vi "Main.vi"() -> ()   [LabVIEW 2017]
uses:
  <vilib>/Utility/file.llb/Write Delimited Spreadsheet (string).vi
  TCP/TCP Engine/SubVIs/SubVI - Global.vi
  TCP/TCP Engine/Controls/RT- Queue States.ctl
  TCP/TCP Engine/TCP/TCP - Driver Control.ctl
  TCP/TCP Engine/TCP/TCP - Signal Names.ctl
  TCP/TCP Engine/TCP/TCP - Signals.ctl
  Global_simulator.vi
panel:
  out "Datalog Interval":dbl
  out "Test Running":bool
  out "Elapsed Time":dbl format="%#.2g"
  out "File Path":path
  out "Test Running":bool
  out "Test Start":u32
  in  "error in (no error)":errorcluster
  out "Data 2":u32
  out "Data 1":u32
  in  "DI 64":bool
  in  "DI 63":bool
  in  "DI 62":bool
  in  "DI 61":bool
  in  "DI 60":bool
  in  "DI 59":bool
  in  "DI 58":bool
  in  "DI 57":bool
  in  "DI 56":bool
  in  "DI 55":bool
  in  "DI 54":bool
  in  "DI 53":bool
  in  "DI 52":bool
  in  "DI 51":bool
  in  "DI 50":bool
  in  "DI 49":bool
  in  "DI 48":bool
  in  "DI 47":bool
  in  "DI 46":bool
  in  "DI 45":bool
  in  "DI 44":bool
  in  "DI 43":bool
  in  "DI 42":bool
  in  "DI 41":bool
  in  "DI 40":bool
  in  "DI 39":bool
  in  "DI 38":bool
  in  "DI 37":bool
  in  "DI 36":bool
  in  "DI 35":bool
  in  "DI 34":bool
  in  "DI 33":bool
  in  "DI 32":bool
  in  "DI 31":bool
  in  "DI 30":bool
  in  "DI 29":bool
  in  "DI 28":bool
  in  "DI 27":bool
  in  "DI 26":bool
  in  "DI 25":bool
  in  "DI 24":bool
  in  "DI 23":bool
  in  "DI 22":bool
  in  "DI 21":bool
  in  "DI 20":bool
  in  "DI 19":bool
  in  "DI 18":bool
  in  "DI 17":bool
  in  "DI 16":bool
  in  "DI 15":bool
  in  "DI 14":bool
  in  "DI 13":bool
  in  "DI 12":bool
  in  "DI 11":bool
  in  "DI 10":bool
  in  "DI 9":bool
  in  "DI 8":bool
  in  "DI 7":bool
  in  "DI 6":bool
  in  "DI 5":bool
  in  "DI 4":bool
  in  "DI 3":bool
  in  "DI 2":bool
  in  "DI 1":bool
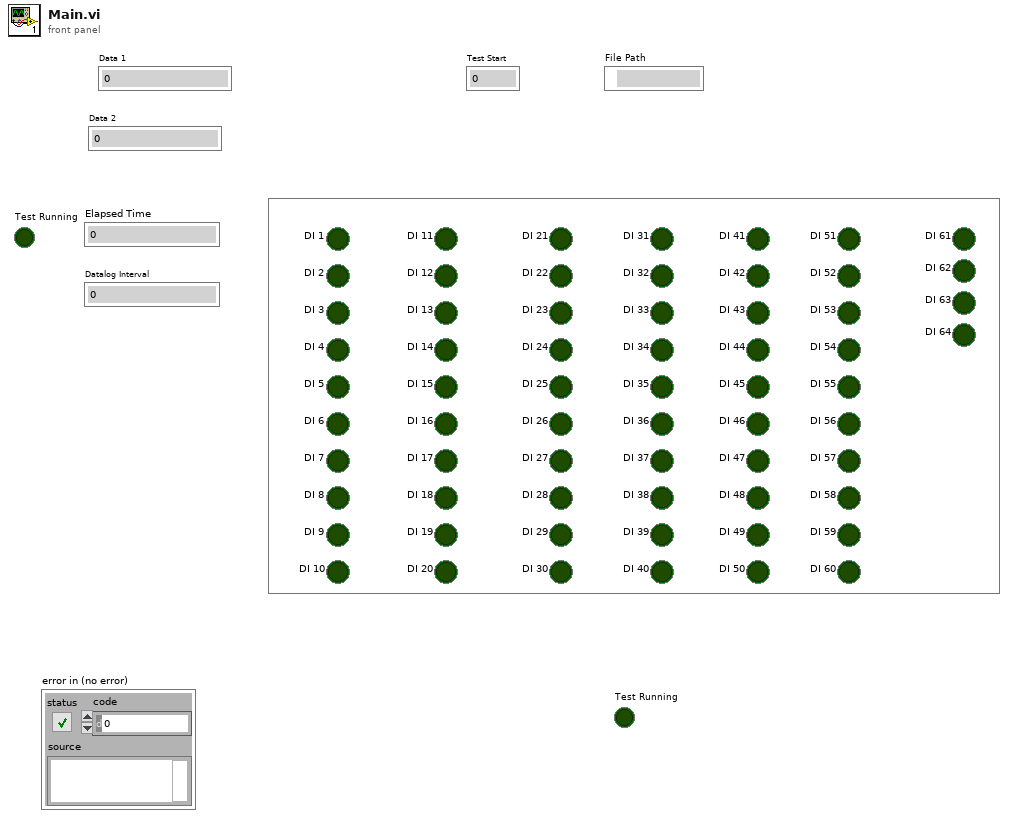
[diagram p1: front panel]
types:
  T1 = cluster{"Data 1":u32, "Data 2":u32, "Boolean Data1":bool[], "Boolean Data 2":bool[]}
  T2 = typedef "TCP - Signals.ctl" = cluster{"Signal":T3, "Value":bool, "Data":variant}
  T3 = typedef "TCP - Signal Names.ctl" = enum16{"Test Running", "Update Sensor Data", "Start Test", "Test Started", "Sequence Complete", "Seuence Aborted", "Abort Test", "Test Settings Updated", "Log Path", "Update Manual Values", "Start Aux Logging", "Aux Log Started", "Stop Aux Logging", "Aux Log Stopped", "Set Dyno Config", "Get PID Values", "Reset Emergency", "Copy Log File", "Download Files", "Send Test Details"}
  T4 = typedef "TCP - Driver Control.ctl" = enum16{"Test Settings", "Boolean Commands", "Test Results", "Send Test Details"}
  T5 = typedef "RT- Queue States.ctl" = enum16{"Initialize", "Enqueue", "Enqueue Priority", "Dequeue", "Flush", "Destroy"}
  T6 = cluster{"Histogram Data":i32[], "Sensor Data":i32[], "File Path":path}
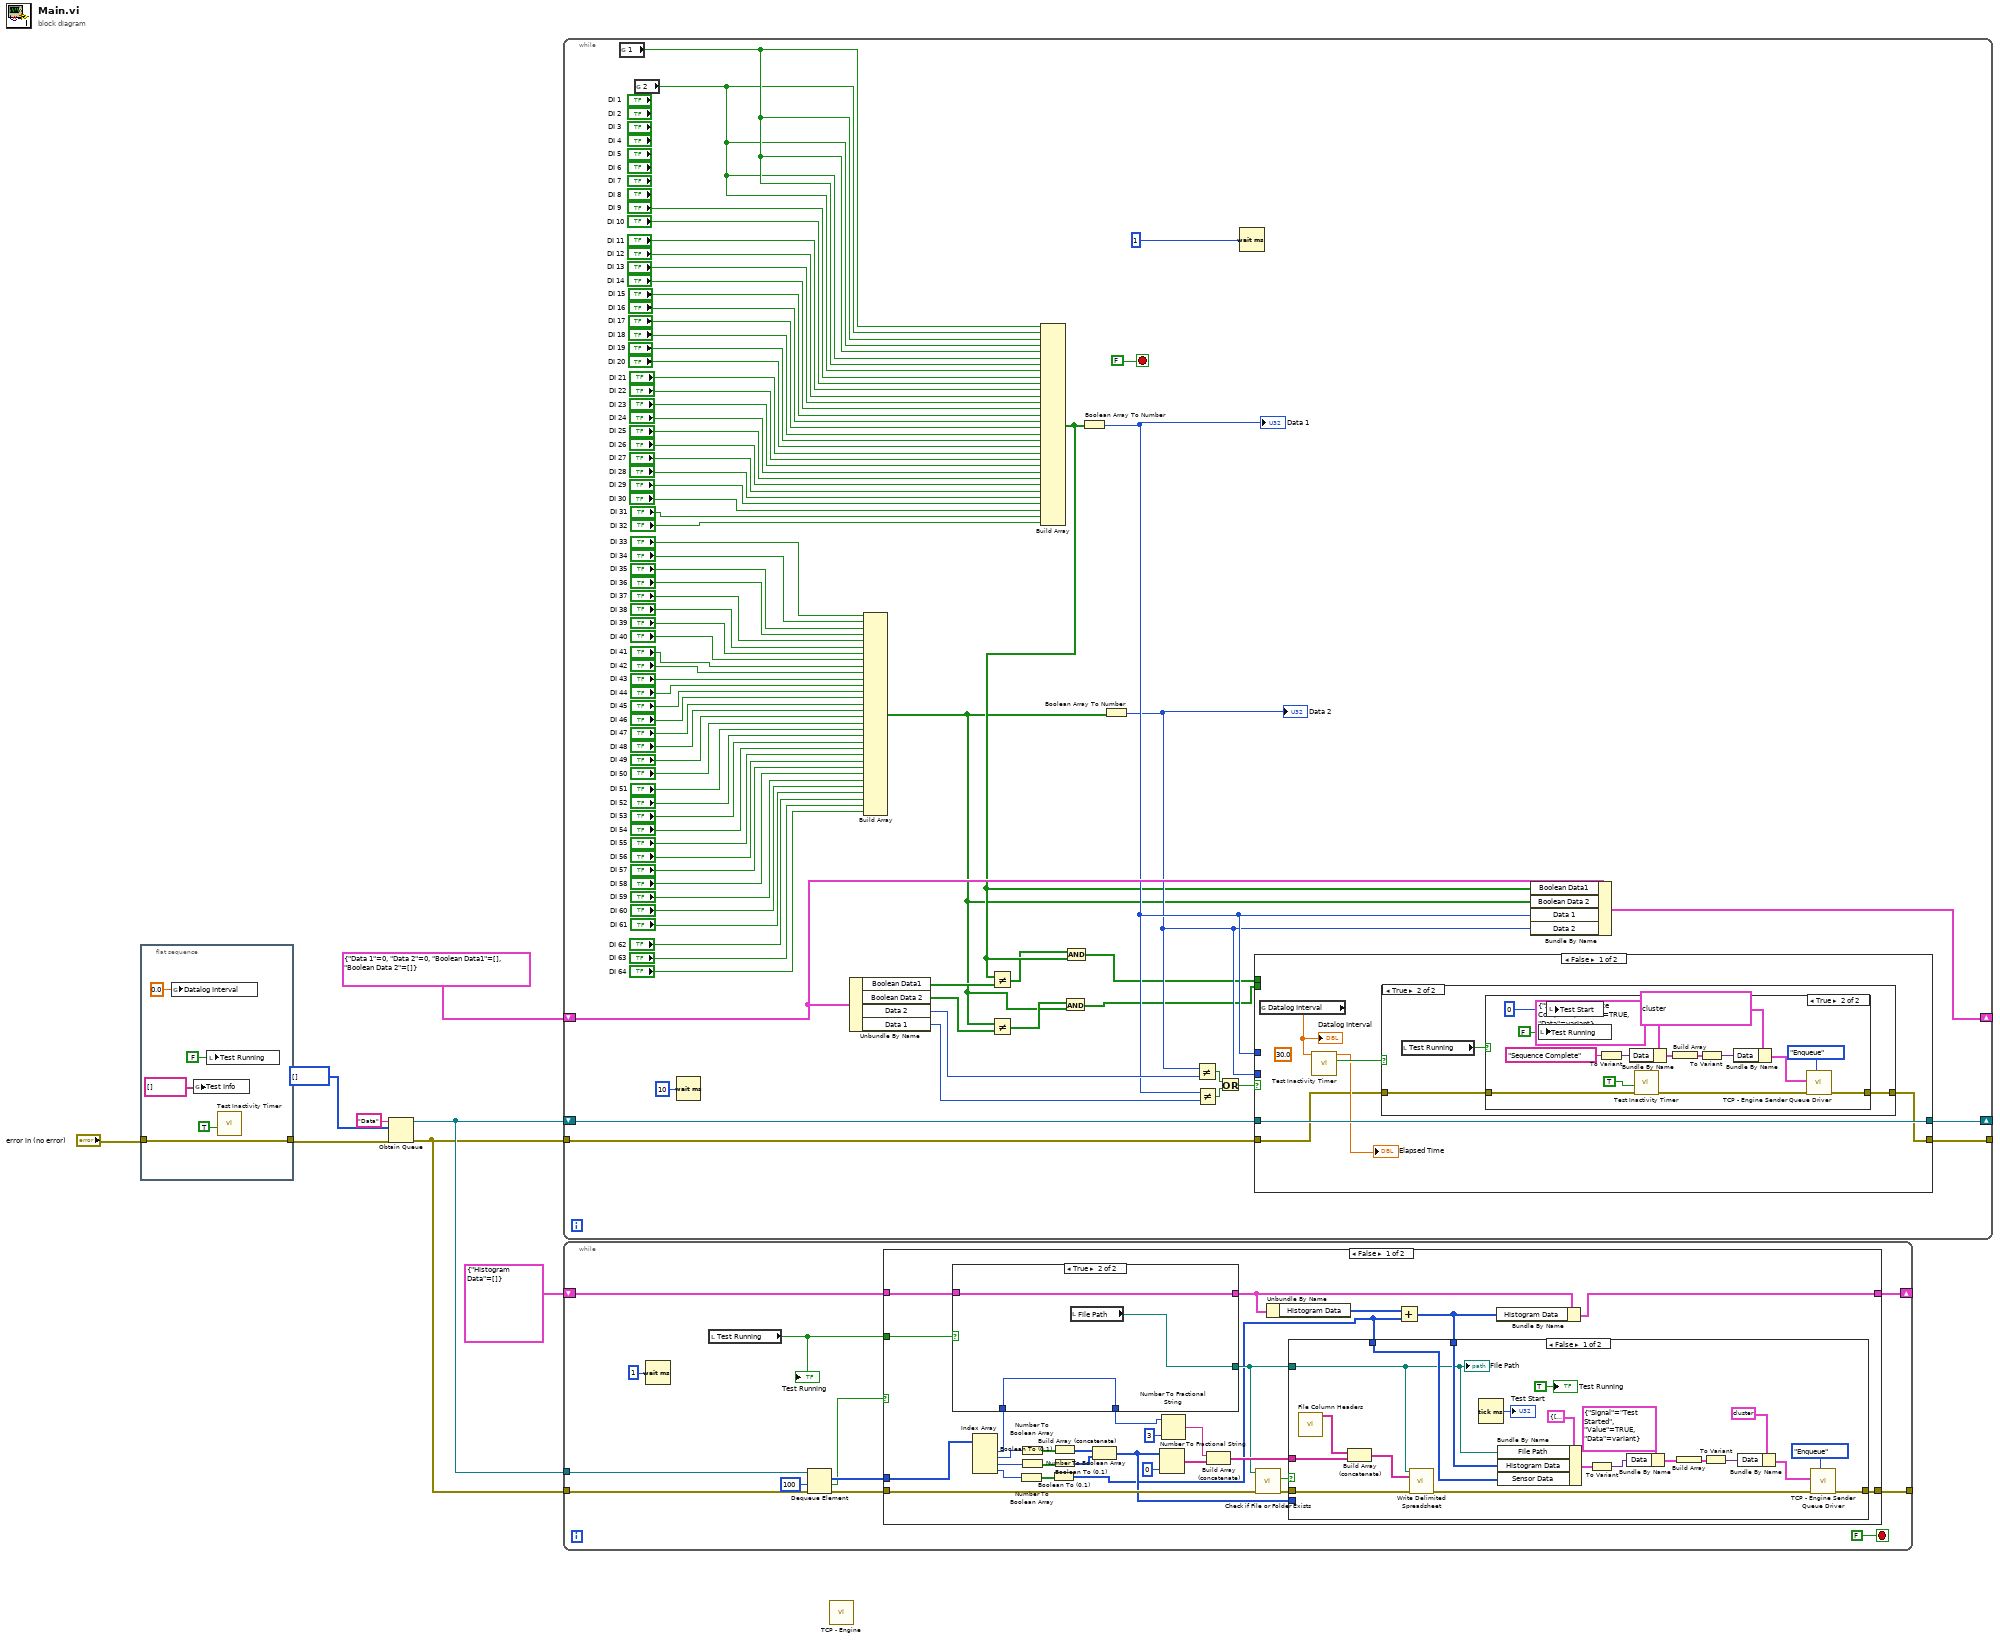
[diagram p0: block diagram]
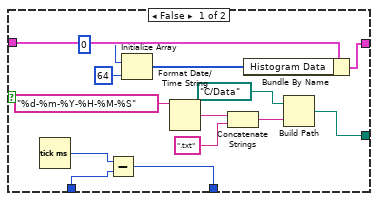
[diagram p2: hidden frame]
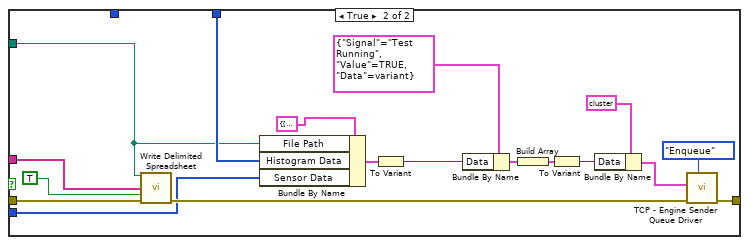
[diagram p3: hidden frame]
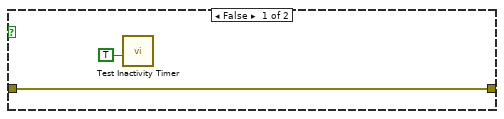
[diagram p6: hidden frame]
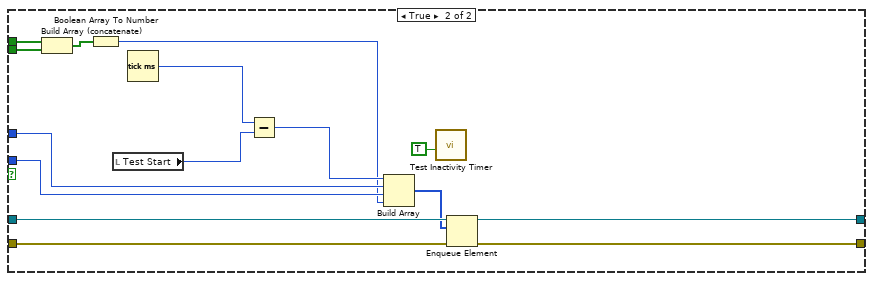
[diagram p7: hidden frame]
diagram:
  n1 = flat-sequence {
    tunnel: [w13] -> w2
    tunnel: "error in (no error)" -> [w13]
    frame #0 {
      n2 = global write "SubVI - Global.vi" "Datalog Interval"(0.0 ("Datalog Interval")) -> ()
      n3 = global write "SubVI - Global.vi" "Test Info"(string[] [] ("Test Info")) -> ()
      n4 = local write "Test Running"(FALSE ("Test Running")) -> ()
      n5 = call "Test Inactivity Timer.vi"("Reset"=TRUE) -> ()  [unwired: 8 in, 3 out]
    }
  }
  n6 = Obtain Queue(name (unnamed)="Data", element data type=u32[] [], error in (no error)=w2) -> (queue out=w5:refnum<queue>, error out=w4:errorcluster)  [unwired: 2 in, 1 out]
  n7 = while {
    shift-right: [w35] -> _
    shift-left: w5 -> [w37]
    tunnel: w4 -> [w36]
    tunnel: [w34] -> _
    shift-right: [w25] -> _
    shift-left: T1 {"Data 1"=0, "Data 2"=0, "Boolean Data1"=[], "Boolean Data 2"=[]} -> [w28]
    stop <- FALSE stop-if-true
    n8 = global read "Global_simulator.vi" "1"() -> (w15:bool)
    n9 = global read "Global_simulator.vi" "2"() -> (w14:bool)
    n10 = Wait (ms)(milliseconds to wait=u32 10) -> ()  [unwired: 1 out]
    n11 = Unbundle By Name(w28) -> ("Boolean Data1"=w23:bool[], "Boolean Data 2"=w22:bool[], "Data 2"=w32:u32, "Data 1"=w33:u32)
    n12 = Build Array("DI 33", "DI 34", "DI 35", "DI 36", "DI 37", "DI 38", "DI 39", "DI 40", "DI 41", "DI 42", "DI 43", "DI 44", "DI 45", "DI 46", "DI 47", "DI 48", "DI 49", "DI 50", "DI 51", "DI 52", "DI 53", "DI 54", "DI 55", "DI 56", "DI 57", "DI 58", "DI 59", "DI 60", "DI 61", "DI 62", "DI 63", "DI 64") -> (w18:bool[])
    n13 = Not Equal?(x=w18, y=w22) -> (x != y?=w21:bool[])
    n14 = Build Array(w15, w14, w15, w14, w15, w14, w15, w14, "DI 9", "DI 10", "DI 11", "DI 12", "DI 13", "DI 14", "DI 15", "DI 16", "DI 17", "DI 18", "DI 19", "DI 20", "DI 21", "DI 22", "DI 23", "DI 24", "DI 25", "DI 26", "DI 27", "DI 28", "DI 29", "DI 30", "DI 31", "DI 32") -> (w19:bool[])
    n15 = Not Equal?(x=w19, y=w23) -> (x != y?=w17:bool[])
    n16 = And(x=w21, y=w18) -> (x .and. y?=w20:bool[])
    n17 = And(x=w17, y=w19) -> (x .and. y?=w16:bool[])
    n18 = Boolean Array To Number(Boolean array=w19) -> (number=w27:u32)
    "Data 1" <- w27
    n19 = Boolean Array To Number(Boolean array=w18) -> (number=w26:u32)
    "Data 2" <- w26
    n20 = Not Equal?(x=w26, y=w32) -> (x != y?=w31:bool)
    n21 = Not Equal?(x=w27, y=w33) -> (x != y?=w30:bool)
    n22 = Or(x=w31, y=w30) -> (x .or. y?=w29:bool)
    n23 = Wait (ms)(milliseconds to wait=u32 1) -> ()  [unwired: 1 out]
    n24 = case shown="False" w29 {
      tunnel: w37 -> [w101 w137]
      tunnel: w36 -> [w97 w136]
      tunnel: [w101 w135] -> w35
      tunnel: [w98 w134] -> w34
      tunnel: w27 -> [_ w130]
      tunnel: w26 -> [_ w129]
      tunnel: w16 -> [_ w126]
      tunnel: w20 -> [_ w125]
      frame False {
        (unwired) 30.0 ("Target Time")
        n25 = global read "SubVI - Global.vi" "Datalog Interval"() -> (w96:dbl)
        "Datalog Interval" <- w96
        n26 = call "Test Inactivity Timer.vi"("Target Time"=w96) -> ("Time Elapsed"=w100:bool, "Elapsed Time"=→"Elapsed Time":dbl)  [unwired: 8 in, 1 out]
        n27 = case shown="True" w100 {
          tunnel: [w102 w105] -> w98
          tunnel: w97 -> [w102 w104]
          frame False {
          }
          frame True {
            n28 = local read "Test Running"() -> (w103:bool)
            n29 = case shown="True" w103 {
              tunnel: [w107 w111] -> w105
              tunnel: w104 -> [w107 w110]
              frame False {
                n30 = call "Test Inactivity Timer.vi"("Reset"=TRUE) -> ()  [unwired: 8 in, 3 out]
              }
              frame True {
                n31 = local write "Test Running"(FALSE ("Test Running")) -> ()
                n32 = local write "Test Start"(u32 0 ("Test Start")) -> ()
                n33 = To Variant(anything="Sequence Complete") -> (Variant=w108:variant)
                n34 = Bundle By Name(cluster=T2 {"Signal"=enum."Sequence Complete", "Value"=TRUE, "Data"=variant}, "Data"=w108) -> (w117:T2)
                n35 = call "Test Inactivity Timer.vi"("error in (no error)"=w110, "Reset"=TRUE) -> ("error out"=w112:errorcluster)  [unwired: 7 in, 2 out]
                n36 = Build Array(w117) -> (w119:T2[])
                n37 = To Variant(anything=w119) -> (Variant=w118:variant)
                n38 = Bundle By Name(cluster=cluster{"Data":variant, "State":T4} {"Data"=variant, "State"=enum."Boolean Commands"} ("Element In"), "Data"=w118) -> (w113:cluster{"Data":variant, "State":T4})
                n39 = call "TCP - Engine Sender Queue Driver.vi"("Cases"=RT-_Queue_States."Enqueue", "error in (no error)"=w112, "Element In"=w113) -> ("error out"=w111:errorcluster)  [unwired: 6 in, 2 out]
              }
            }
          }
        }
      }
      frame True {
        n40 = Build Array (concatenate)(w126, w125) -> (w124:bool[])
        n41 = Boolean Array To Number(Boolean array=w124) -> (number=w123:u32)
        n42 = local read "Test Start"() -> (w127:u32)
        n43 = Tick Count (ms)() -> (millisecond timer value=w128:u32)
        n44 = Subtract(x=w128, y=w127) -> (x-y=w132:u32)
        n45 = Build Array(w132, w130, w129, w123) -> (w133:u32[])
        n46 = call "Test Inactivity Timer.vi"("Reset"=TRUE) -> ()  [unwired: 8 in, 3 out]
        n47 = Enqueue Element(queue=w137, element=w133, error in (no error)=w136) -> (queue out=w135:refnum<queue>, error out=w134:errorcluster)  [unwired: 1 in, 1 out]
      }
    }
    n48 = Bundle By Name(cluster=w28, "Boolean Data1"=w19, "Boolean Data 2"=w18, "Data 1"=w27, "Data 2"=w26) -> (w25:T1)
  }
  n49 = while {
    tunnel: w5 -> [w148]
    tunnel: w4 -> [w147]
    tunnel: [w144] -> _
    shift-right: [w138] -> _
    shift-left: cluster{"Histogram Data":i32[]} {"Histogram Data"=[]} -> [w139]
    stop <- FALSE stop-if-true
    n50 = Wait (ms)(milliseconds to wait=u32 1) -> ()  [unwired: 1 out]
    n51 = local read "Test Running"() -> (w143:bool)
    "Test Running" <- w143
    n52 = Dequeue Element(queue=w148, timeout in ms (-1)=100, error in (no error)=w147) -> (element=w146:u32[], timed out?=w140:bool, error out=w145:errorcluster)  [unwired: 1 out]
    n53 = case shown="False" w140 {
      tunnel: w146 -> [w178 _]
      tunnel: w145 -> [w169 w236]
      tunnel: [w166 w236] -> w144
      tunnel: w143 -> [w163 _]
      tunnel: w139 -> [w162 w235]
      tunnel: [w160 w235] -> w138
      frame False {
        n54 = Index Array(array=w178) -> (element #1=w153:u32, element #2=w177:u32, element #3=w176:u32, element #4=w155:u32)  [unwired: 4 in]
        n55 = case shown="True" w163 {
          tunnel: [w189 w195] -> w164
          tunnel: w162 -> [w186 w194]
          tunnel: [w185 w194] -> w161
          tunnel: w153 -> [w180 w193]
          tunnel: [w179 w193] -> w152
          frame False {
            n56 = Tick Count (ms)() -> (millisecond timer value=w181:u32)
            n57 = Subtract(x=w181, y=w180) -> (x-y=w179:u32)
            n58 = Initialize Array(0 ("Histogram Data"), 64 ("dimension size")) -> (w182:i32[])
            n59 = Format Date/Time String(time format string (%c)="%d-%m-%Y-%H-%M-%S") -> (date/time string=w190:string)  [unwired: 2 in]
            n60 = Concatenate Strings(w190, ".txt" ("string")) -> (w188:string)
            n61 = Bundle By Name(cluster=w186, "Histogram Data"=w182) -> (w185:cluster{"Histogram Data":i32[]})
            n62 = Build Path(base path=path "C:/Data", name or relative path=w188) -> (appended path=w189:path)
          }
          frame True {
            n63 = local read "File Path"() -> (w195:path)
          }
        }
        n64 = Number To Boolean Array(number=w155) -> (Boolean array=w156:bool[])
        n65 = Number To Boolean Array(number=w177) -> (Boolean array=w175:bool[])
        n66 = Number To Boolean Array(number=w176) -> (Boolean array=w174:bool[])
        n67 = Boolean To (0,1)(Boolean=w156) -> (0, 1=w154:i16[])
        n68 = Boolean To (0,1)(Boolean=w175) -> (0, 1=w173:i16[])
        n69 = Boolean To (0,1)(Boolean=w174) -> (0, 1=w172:i16[])
        n70 = Build Array (concatenate)(w173, w172) -> (w157:i16[])
        n71 = Number To Fractional String(number=w157, precision (6)=i16 0) -> (F-format string=w170:string[])  [unwired: 2 in]
        n72 = Number To Fractional String(number=w152, precision (6)=i16 3) -> (F-format string=w150:string)  [unwired: 2 in]
        n73 = Build Array (concatenate)(w150, w170) -> (w165:string[])
        n74 = call <vilib>:"Check if File or Folder Exists.vi"("error in (no error)"=w169, "path"=w164) -> ("error out"=w168:errorcluster, "file or folder exists?"=w167:bool)  [unwired: 7 in, 1 out]
        n75 = Unbundle By Name(w161) -> ("Histogram Data"=w159:i32[])
        n76 = Add(x=w159, y=w154) -> (x+y=w158:i32[])
        n77 = case shown="False" w167 {
          tunnel: w165 -> [w215 w234]
          tunnel: w164 -> [w196 w218]
          tunnel: w168 -> [w213 w232]
          tunnel: [w202 w223] -> w166
          tunnel: w157 -> [_ w217]
          tunnel: w158 -> [w199 w221]
          tunnel: w154 -> [w198 _]
          frame False {
            n78 = call "File Column Headers.vi"() -> ("Column Header"=w216:string[][])  [unwired: 11 in]
            n79 = Build Array (concatenate)(w216, w215) -> (w214:string[][])
            n80 = call-poly <vilib>:"Write Delimited Spreadsheet.vi"("file path (dialog if empty)"=w196, "2D data"=w214, "error in (no error)"=w213) -> ("error out"=w203:errorcluster)  [unwired: 11 in, 1 out]
            n81 = Tick Count (ms)() -> (millisecond timer value=→"Test Start":u32)
            n82 = Bundle By Name(cluster=T6 {"Histogram Data"=[], "Sensor Data"=[], "File Path"=path ""}, "File Path"=w196, "Histogram Data"=w199, "Sensor Data"=w198) -> (w197:T6)
            n83 = To Variant(anything=w197) -> (Variant=w206:variant)
            n84 = Bundle By Name(cluster=T2 {"Signal"=enum."Test Started", "Value"=TRUE, "Data"=variant}, "Data"=w206) -> (w205:T2)
            n85 = Build Array(w205) -> (w201:T2[])
            n86 = To Variant(anything=w201) -> (Variant=w204:variant)
            n87 = Bundle By Name(cluster=cluster{"Data":variant, "State":T4} {"Data"=variant, "State"=enum."Boolean Commands"} ("Element In"), "Data"=w204) -> (w208:cluster{"Data":variant, "State":T4})
            n88 = call "TCP - Engine Sender Queue Driver.vi"("Cases"=RT-_Queue_States."Enqueue", "error in (no error)"=w203, "Element In"=w208) -> ("error out"=w202:errorcluster)  [unwired: 6 in, 2 out]
            "Test Running" <- TRUE ("Test Running")
            "File Path" <- w196
          }
          frame True {
            n89 = call-poly <vilib>:"Write Delimited Spreadsheet.vi"("file path (dialog if empty)"=w218, "1D data"=w234, "append to file? (new file:F)"=TRUE, "error in (no error)"=w232) -> ("error out"=w224:errorcluster)  [unwired: 10 in, 1 out]
            n90 = Bundle By Name(cluster=T6 {"Histogram Data"=[], "Sensor Data"=[], "File Path"=path ""}, "File Path"=w218, "Histogram Data"=w221, "Sensor Data"=w217) -> (w222:T6)
            n91 = To Variant(anything=w222) -> (Variant=w220:variant)
            n92 = Bundle By Name(cluster=T2 {"Signal"=enum."Test Running", "Value"=TRUE, "Data"=variant}, "Data"=w220) -> (w227:T2)
            n93 = Build Array(w227) -> (w225:T2[])
            n94 = To Variant(anything=w225) -> (Variant=w226:variant)
            n95 = Bundle By Name(cluster=cluster{"Data":variant, "State":T4} {"Data"=variant, "State"=enum."Boolean Commands"} ("Element In"), "Data"=w226) -> (w229:cluster{"Data":variant, "State":T4})
            n96 = call "TCP - Engine Sender Queue Driver.vi"("Cases"=RT-_Queue_States."Enqueue", "error in (no error)"=w224, "Element In"=w229) -> ("error out"=w223:errorcluster)  [unwired: 6 in, 2 out]
          }
        }
        n97 = Bundle By Name(cluster=w161, "Histogram Data"=w158) -> (w160:cluster{"Histogram Data":i32[]})
      }
      frame True {
      }
    }
  }
  n98 = call "TCP - Engine.vi"() -> ()  [unwired: 12 in]
